vi "solar_write QTimerAdd.vi"(8 "error in (no error)":errorcluster, 10 "QTimer Settings":T1={"QTimer"="", "Delay"=0, "Start"=FALSE, "EnQ_Type"=enum."IgnoreIfExists", "Messages"=[]}, 11 "solar in":refnum<class "solar.lvclass">) -> (0 "error out":errorcluster, 3 "solar out":refnum<class "solar.lvclass">)   [LabVIEW 2018, in "solar.lvclass"]
doc: "This launches a QTimer daemon to enqueue to this target's queue. If the QTimer already exists, this only sets the QTimer settings."
uses:
  solar.lvclass
  qtimer/solar_qtimer_ctl QTimer Settings.ctl
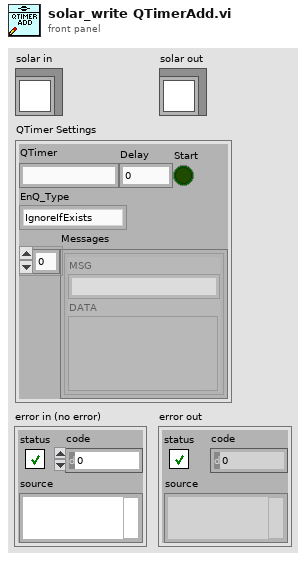
[diagram p1: front panel]
types:
  T1 = typedef "solar_qtimer_ctl QTimer Settings.ctl" = cluster{"QTimer":string, "Delay":i32, "Start":bool, "EnQ_Type":enum8{"Normal", "Priority", "IgnoreIfExists"}, "Messages":cluster{"MSG":string, "DATA":variant}[]}
  T2 = typedef "solar_ctl SOLAR Refnum.ctl" = refnum<k1>
  T3 = typedef "solar_ctl SOLAR Global.ctl" = cluster{"Targets":T4[], "AppDir":path, "solar.ini":path, "ConfigsDir":path, "CosmosDir":path, "LogsDir":path, "ExePath":path, "ExeVersion":string, "PartNum":string, "AppSetup":string, "Title":string, "Main.ini":path, "Temp.ini":path, "vSOLAR":string, "Splash.png":string, "SplashWait":i32, "SOLARUE":refnum<user-event>, "VoyagerRefnum":T5, "QTimerRefnum":T6}
  T4 = typedef "solar_ctl Target Global.ctl" = cluster{"Target":string, "Q":refnum<queue>, "UE":refnum<user-event>, "VI":refnum<vi>, "Menu":refnum<k9>, "Data":refnum<data-value>, "Attributes":variant}
  T5 = typedef "solar_voy_ctl Voyager Refnum.ctl" = refnum<k1>
  T6 = typedef "solar_qtimer_ctl Refnum.ctl" = refnum<k1>
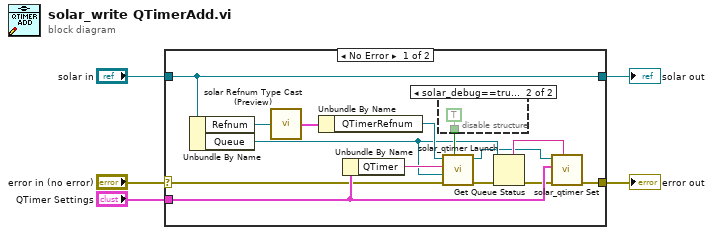
[diagram p0: block diagram]
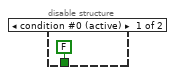
[diagram p2: hidden frame]
diagram:
  n1 = case shown="No Error" "error in (no error)" {
    selector: "error in (no error)" -> [w9 w23]
    tunnel: "solar in" -> [w17 w22]
    tunnel: [w14 w23] -> w4
    tunnel: [w17 w22] -> w2
    tunnel: "QTimer Settings" -> [w13 _]
    frame No Error {
      n2 = Unbundle By Name(w17) -> ("Refnum"=w19:T2, "Queue"=w11:refnum<queue>)
      n3 = call "solar Refnum Type Cast (Preview).vi"("Refnum"=w19) -> ("SOLAR"=w18:T3)  [unwired: 8 in]
      n4 = Unbundle By Name(w18) -> ("QTimerRefnum"=w16:T6)
      n5 = Unbundle By Name(w13) -> ("QTimer"=w15:string)
      n6 = disable-structure shown="solar_debug==true" {
        disable-tunnel: [FALSE TRUE ("Open FP? (F)")] -> w12
        frame condition #0 (active) {
        }
        frame condition #1 {
        }
      }
      n7 = call "solar_qtimer Launch.vi"("Open FP? (F)"=w12, "error in (no error)"=w9, "Target Queue"=w11, "QTimer Name"=w15, "QTimer Refnum in"=w16) -> ("error out"=w8:errorcluster, "QTimer Refnum out"=w6:T6)  [unwired: 5 in]
      n8 = Get Queue Status(queue=w11, error in (no error)=w8) -> (queue name=w10:string, error out=w7:errorcluster)  [unwired: 1 in, 6 out]
      n9 = call "solar_qtimer Set.vi"("Target Name"=w10, "error in (no error)"=w7, "Settings"=w13, "QTimer Refnum in"=w6) -> ("error out"=w14:errorcluster)  [unwired: 6 in, 1 out]
    }
    frame Error {
    }
  }
  "error out" <- w4
  "solar out" <- w2
